vi "Sabertooths in use gvar.vi"() -> ()   [LabVIEW 2018]
uses:
  controls/All Addresses.ctl
panel:
  out "All Addresses":T1
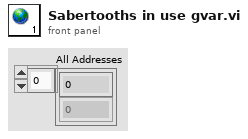
[diagram p1: front panel]
types:
  T1 = typedef "All Addresses.ctl" = u8[]
diagram:
